vi "GetClassAttribute1.vi"(5 "error in (no error)":errorcluster) -> (15 "Int":i32, 16 "ArrayInt":i32[](array[numeric]), 17 "SubClassIntAttribute":i32, 19 "error out":errorcluster)   [LabVIEW 2010, in "G#SubClass1.lvclass"]
uses:
  G#SubClass1.lvclass
  G#BaseClass1_class/G#BaseClass1.lvclass
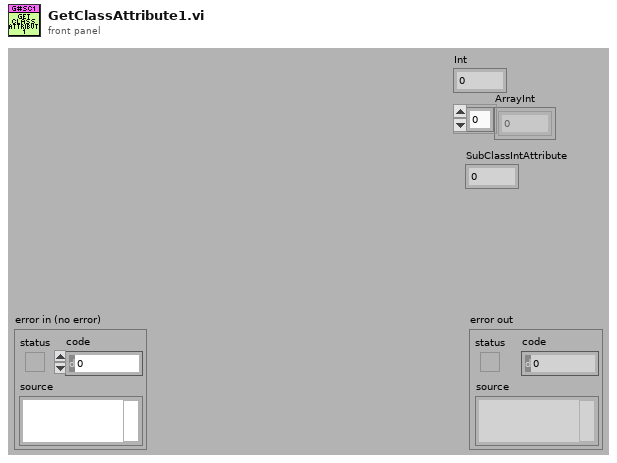
[diagram p1: front panel]
types:
  T1 = typedef "G#SubClass1.lvclass/ClassAttributes.ctl" = cluster{"SubClassIntAttribute":i32}
  T2 = typedef "G#BaseClass1.lvclass/ClassAttributes.ctl" = cluster{"Int":i32, "ArrayInt":i32[]}
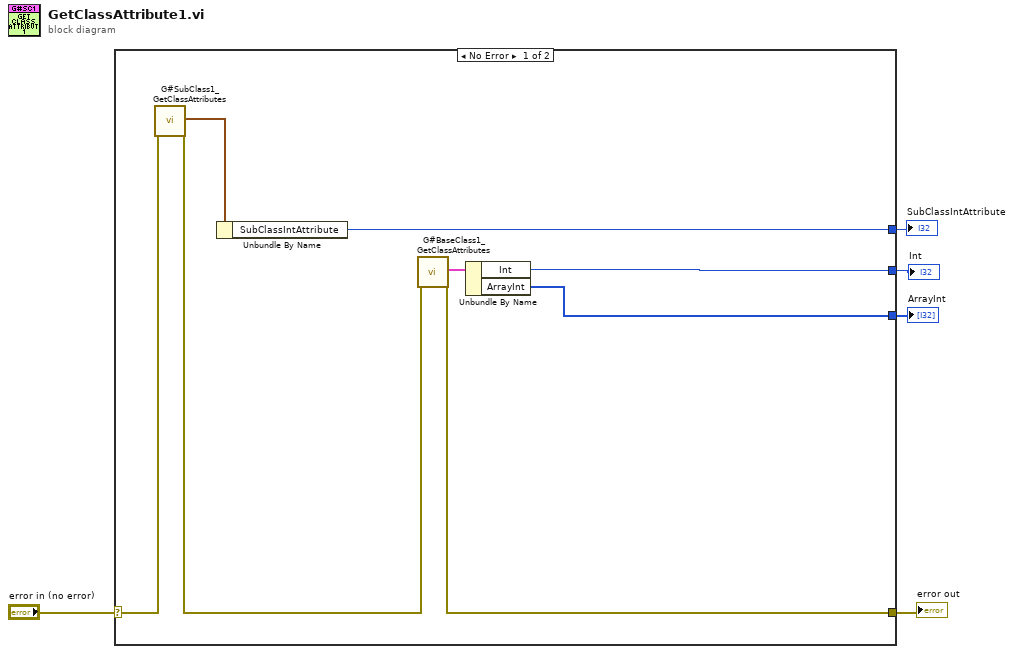
[diagram p0: block diagram]
diagram:
  n1 = case shown="No Error" "error in (no error)" {
    selector: "error in (no error)" -> [w13 w14]
    tunnel: [w9 w14] -> w4
    tunnel: [w11 _] -> w3
    tunnel: [w7 _] -> w2
    tunnel: [w6 _] -> w1
    frame No Error {
      n2 = call "G#SubClass1_GetClassAttributes.vi"("error in (no error)"=w13) -> ("class attributes"=w12:T1, "error out"=w10:errorcluster)  [unwired: 15 in, 2 out]
      n3 = Unbundle By Name(w12) -> ("SubClassIntAttribute"=w11:i32)
      n4 = call "G#BaseClass1_GetClassAttributes.vi"("error in (no error)"=w10) -> ("class attributes"=w8:T2, "error out"=w9:errorcluster)  [unwired: 15 in, 2 out]
      n5 = Unbundle By Name(w8) -> ("Int"=w7:i32, "ArrayInt"=w6:i32[])
    }
    frame Error {
    }
  }
  "error out" <- w4
  "Int" <- w2
  "ArrayInt" <- w1
  "SubClassIntAttribute" <- w3
